vi "VDA Stop DAC.vi"(8 "error in (no error)":errorcluster, 9 "Channel":u8, 10 "DevIndex":i32, 11 "DevType":i32) -> (0 "error out":errorcluster, 3 "function return":i32)   [LabVIEW 2010, in "CntrolDAC.lvlib"]
doc: "int WINAPI VDA_StopDAC(int DevType, int DevIndex, unsigned char Channel);"
uses:
  CntrolDAC.lvlib
  labview_32bit/ControlDAC/Ginkgo_Driver.dll
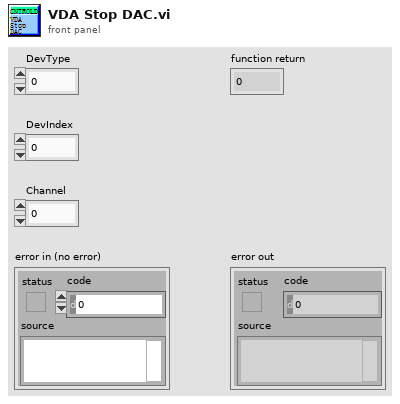
[diagram p1: front panel]
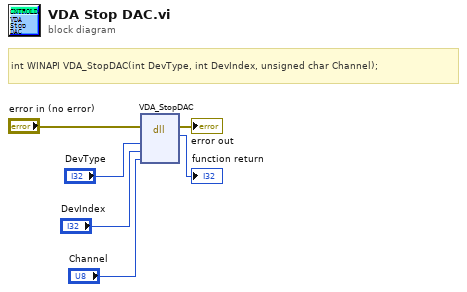
[diagram p0: block diagram]
diagram:
  # "int WINAPI VDA_StopDAC(int DevType, int DevIndex, unsigned char Channel);"
  n1 = dll-call lib="E:/Project/vt_ginkgo/truck/Ginkgo Driver/vs2010/Ginkgo_USB-I2C&SPI&CAN_API_v2.0.3.3/lib/labview_32bit/ControlDAC/Ginkgo_Driver.*" fn="VDA_StopDAC"(error in="error in (no error)", "DevType"="DevType", "DevIndex"="DevIndex", "Channel"="Channel") -> (error out=→"error out":errorcluster, →"function return":i32)  [unwired: 5 in, 1 out]
